vi "Run Test (Object).vi"(4 "timeout (2000 ms)":i32=2000, 5 "Test Report":refnum<class "Test Report.lvclass">, 6 "Verbose":bool, 7 "Report Path":path, 8 "error in":errorcluster, 10 "Object":refnum<class>, 11 "Interactive (T)":bool=TRUE) -> (0 "error out":errorcluster)   [LabVIEW 2013, in "Caraya.lvlib"]
uses:
  Caraya.lvlib
  classes/Test Report/Test Report.lvclass
  classes/Test Runner/Test Runner.lvclass
  classes/Test Runner.Class/Test Runner.Class.lvclass
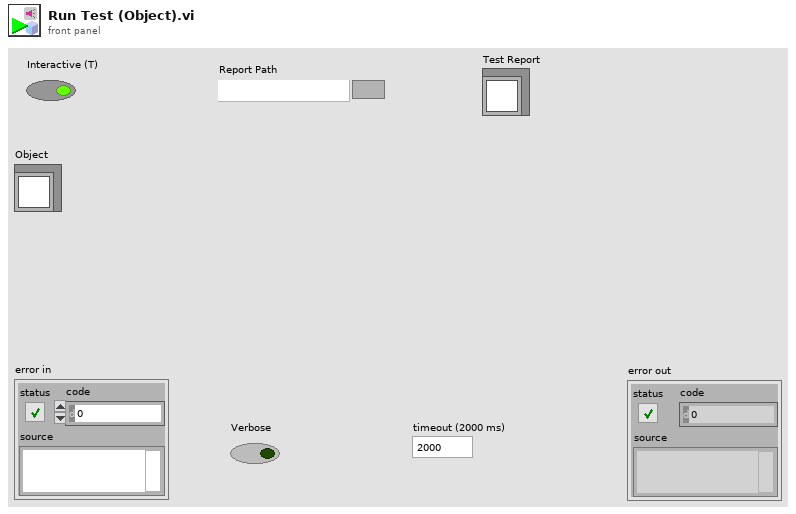
[diagram p1: front panel]
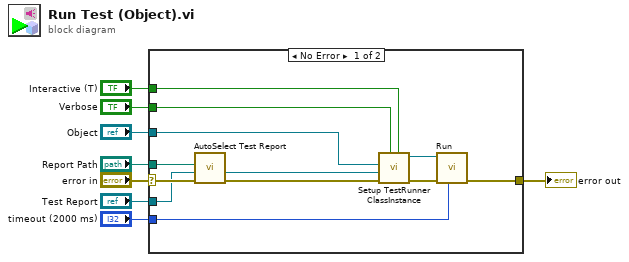
[diagram p0: block diagram]
diagram:
  n1 = case shown="No Error" "error in" {
    selector: "error in" -> [w19 w21]
    tunnel: [w20 w21] -> w8
    tunnel: "Verbose" -> [w13 _]
    tunnel: "Interactive (T)" -> [w12 _]
    tunnel: "Test Report" -> [w17 _]
    tunnel: "Object" -> [w14 _]
    tunnel: "Report Path" -> [w18 _]
    tunnel: "timeout (2000 ms)" -> [w9 _]
    frame No Error {
      n2 = call "AutoSelect Test Report.vi"("error in (no error)"=w19, "Test Report in"=w17, "Report Path"=w18) -> ("error out"=w16:errorcluster, "Test Report out"=w15:refnum<class "Test Report.lvclass">)  [unwired: 7 in]
      n3 = call "Setup TestRunner ClassInstance.vi"("Interactive (T)"=w12, "Verbose (F)"=w13, "error in (no error)"=w16, "Test Report"=w15, "Instance"=w14) -> ("error out"=w11:errorcluster, "Test Runner.Class out"=w10:refnum<class "Test Runner.Class.lvclass">)  [unwired: 5 in]
      n4 = call "Run.vi"("timeout"=w9, "error in (no error)"=w11, "Test Runner in"=w10) -> ("error out"=w20:errorcluster)  [unwired: 7 in, 1 out]
    }
    frame Error {
    }
  }
  "error out" <- w8
